vi "Set Is WebSocket.vi"(10 "Is WebSocket":bool, 11 "Processing in":refnum<class "Processing.lvclass">) -> (3 "Processing out":refnum<class "Processing.lvclass">)   [LabVIEW 2020, in "HTTP Server.lvlib" / "Processing.lvclass"]
uses:
  Processing.lvclass
  Processing.lvclass/Processing.ctl
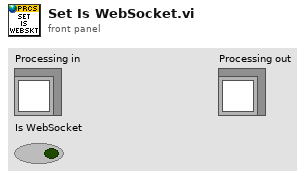
[diagram p1: front panel]
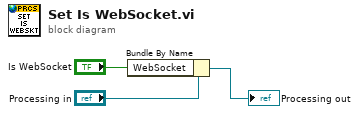
[diagram p0: block diagram]
diagram:
  n1 = Bundle By Name(cluster="Processing in", "WebSocket"="Is WebSocket") -> (→"Processing out":refnum<class "Processing.lvclass">)
